vi "Insert Case Structure.vi"(0 "Custom Type Test Executive in":refnum<class "Custom Type Test Executive.lvclass">, 1 "Name":string, 2 "Unique ID":string, 3 "Insertion Index":i32=-1, 4 "Assertions":refnum<class "Assert.lvclass">[](array[class]), 5 "error in (no error)":errorcluster, 6 "Parent ID":string, 7 "X Variables":string[](array[string]), 9 "Y Variables":string[](array[string]), 11 "Conditional Branches":string[](array[string]), 13 "\"Else\" Conditional Branch":string) -> (12 "Unique ID out":string, 14 "Custom Type Test Executive out":refnum<class "Custom Type Test Executive.lvclass">, 17 "Replaced?":bool, 19 "error out":errorcluster)   [LabVIEW 2017, in "Custom Type Test Executive.lvlib" / "Custom Type Test Executive.lvclass"]
uses:
  <vilib>/gpm_packages/@cs/test-executive/Source/Custom Type Test Executive/Custom Type Test Executive/Custom Type Test Executive.lvclass
  C:/Program Files/National Instruments/LabVIEW 2017/vi.lib/gpm_packages/@cs/test-executive/Source/Test Executive/TestExecutive/Test Executive.lvclass
  <vilib>/gpm_packages/@cs/run-time-assertions/Source/Assert/Assert.lvclass
  <vilib>/gpm_packages/@cs/test-executive/Source/Custom Type Test Executive/Case Structure/Case Structure.lvclass
  <vilib>/gpm_packages/@cs/data-type-serializer/source/I32/I32.lvclass/I32.ctl
  <vilib>/gpm_packages/@cs/data-type-serializer/source/Boolean/Boolean.lvclass/Boolean.ctl
  <vilib>/gpm_packages/@cs/test-executive/Source/Test Executive/TestExecutive/Test Executive.lvclass/Test Executive.ctl
  <vilib>/gpm_packages/@cs/data-type-serializer/source/String 1D/String 1D.lvclass/String 1D.ctl
  <vilib>/gpm_packages/@cs/data-type-serializer/source/Assertion 1D/Assertion 1D.lvclass/Assertion 1D.ctl
  <vilib>/gpm_packages/@cs/data-type-serializer/source/String/String.lvclass/String.ctl
  a9862942-6bcc-4297-8062-ded843aa0e3e.vi
  f111b730-334b-4c51-af02-4347af488b46.vi
  cb5dc6a4-4407-49fc-b22c-1a23020fa038.vi
  5ed2cf76-4d61-4079-ad61-c8732e7cce71.vi
  5ea85d52-ce01-4b8a-819c-f0f3d244220a.vi
  3dbbcc80-fe4b-4aaf-9db7-d8ec31dae2ca.vi
  8353aa7f-a856-40a3-8e40-fb73858b1775.vi
  <vilib>/gpm_packages/@cs/data-type-serializer/source/String 1D/String 1D.lvclass
  <vilib>/gpm_packages/@cs/data-type-serializer/source/Assertion 1D/Assertion 1D.lvclass
  <vilib>/gpm_packages/@cs/data-type-serializer/source/String/String.lvclass
  <vilib>/gpm_packages/@cs/data-type-serializer/source/Boolean/Boolean.lvclass
  <vilib>/gpm_packages/@cs/data-type-serializer/source/I32/I32.lvclass
  <vilib>/gpm_packages/@cs/linked-list/Source/Linked List/ILinkedList/ILinked List.lvclass
  <vilib>/gpm_packages/@cs/linked-list/Source/Linked List/Linked List Ref/Linked List Ref.lvclass
  <vilib>/gpm_packages/@cs/test-executive/Source/Test Executive/TestExecutive/Test Executive.lvclass
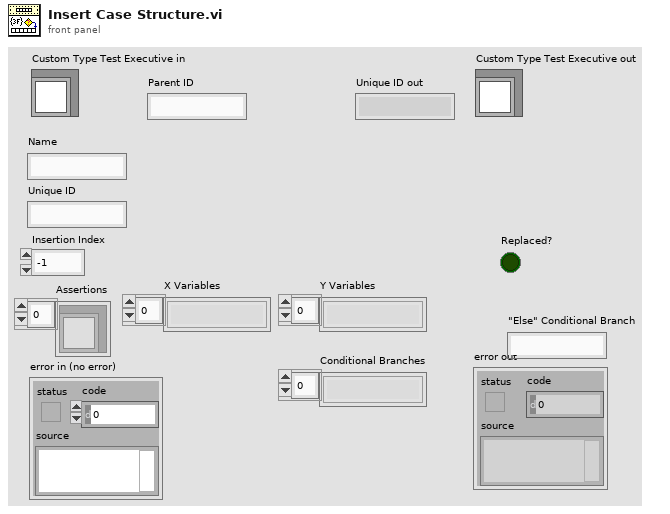
[diagram p1: front panel]
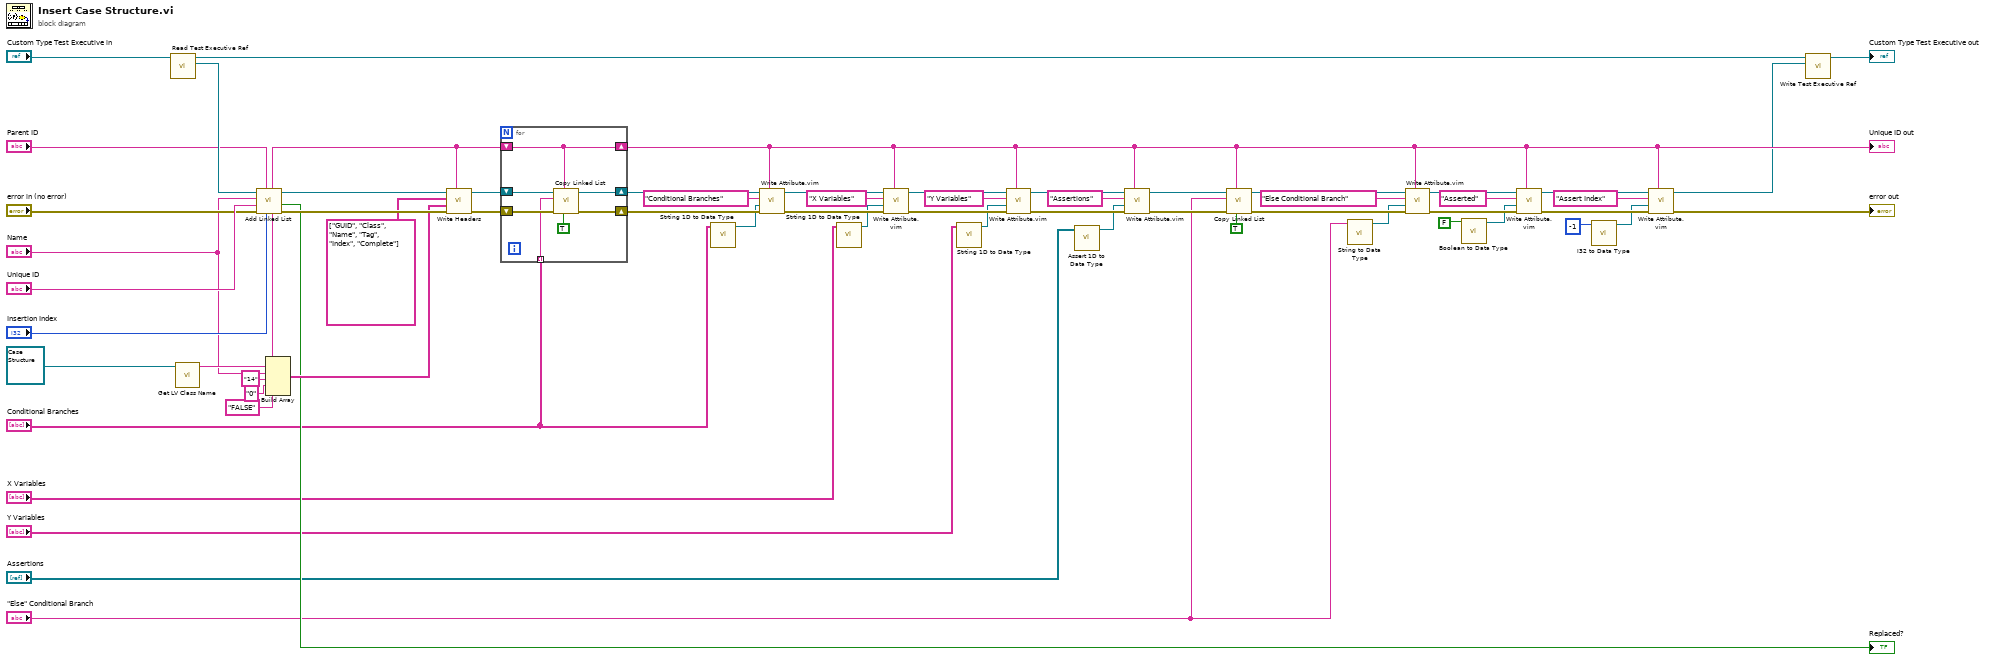
[diagram p0: block diagram]
diagram:
  n1 = call <vilib>:"Read Test Executive Ref.vi"("Test Executive in"="Custom Type Test Executive in") -> ("Test Executive Ref"=w24:refnum<data-value>, "Test Executive out"=w23:refnum<class "Custom Type Test Executive.lvclass">)  [unwired: 9 in]
  n2 = call <vilib>:"Get LV Class Name.vi"("object"=refnum<class "Case Structure.lvclass"> refnum ("Custom Type Test Executive.lvlib:Case Structure.lvclass")) -> ("class name"=w60:string)  [unwired: 9 in, 1 out]
  n3 = call <vilib>:"Add Linked List.vi"("Insertion Index"="Insertion Index", "Parent ID"="Parent ID", "error in (no error)"="error in (no error)", "Linked List ID"="Unique ID", "Name"="Name", "Linked List Ref"=w24) -> ("error out"=w62:errorcluster, "Replaced?"=→"Replaced?":bool, "Linked List Ref out"=w63:refnum<data-value>, "Linked List ID out"=w41:string)  [unwired: 2 in]
  n4 = Build Array(w41, w60, "Name", "14" ("element"), "0" ("element"), "FALSE" ("element")) -> (w58:string[])
  n5 = call <vilib>:"Write Headers.vi"("Linked List ID"=w41, "error in (no error)"=w62, "Header Values"=w58, "Header Names"=string[] ["GUID", "Class", "Name", "Tag", "Index", "Complete"], "Linked List Ref"=w63) -> ("error out"=w56:errorcluster, "Linked List Ref out"=w57:refnum<data-value>)  [unwired: 5 in]
  n6 = for {
    tunnel: "Conditional Branches" -> [w65] mode=indexing
    shift-right: [w67] -> w40
    shift-left: w57 -> [w70]
    shift-right: [w66] -> w39
    shift-left: w56 -> [w69]
    shift-right: [w64] -> w27
    shift-left: w41 -> [w64]
    n7 = call <vilib>:"Copy Linked List.vi"("Move?"=TRUE, "New Parent Linked List ID"=w64, "error in (no error)"=w69, "Linked List ID"=w65, "Linked List Ref"=w70) -> ("error out"=w66:errorcluster, "Linked List Ref out"=w67:refnum<data-value>)  [unwired: 3 in, 2 out]
  }
  "Unique ID out" <- w27
  n8 = call <vilib>:"Strting 1D to Data Type.vi"("String 1D"="Conditional Branches") -> ("Boolean out"=w13:refnum<class "String 1D.lvclass">)  [unwired: 9 in, 1 out]
  n9 = call "Write Attribute.vim"("Linked List ID"=w27, "error in (no error)"=w39, "Attribute"=w13, "Attribute Name"="Conditional Branches", "Linked List Ref"=w40) -> ("error out"=w37:errorcluster, "Linked List Ref out"=w38:refnum<data-value>)  [unwired: 3 in, 2 out]
  n10 = call <vilib>:"Strting 1D to Data Type.vi"("String 1D"="X Variables") -> ("Boolean out"=w11:refnum<class "String 1D.lvclass">)  [unwired: 9 in, 1 out]
  n11 = call "Write Attribute.vim"("Linked List ID"=w27, "error in (no error)"=w37, "Attribute"=w11, "Attribute Name"="X Variables", "Linked List Ref"=w38) -> ("error out"=w52:errorcluster, "Linked List Ref out"=w53:refnum<data-value>)  [unwired: 3 in, 2 out]
  n12 = call <vilib>:"Strting 1D to Data Type.vi"("String 1D"="Y Variables") -> ("Boolean out"=w9:refnum<class "String 1D.lvclass">)  [unwired: 9 in, 1 out]
  n13 = call "Write Attribute.vim"("Linked List ID"=w27, "error in (no error)"=w52, "Attribute"=w9, "Attribute Name"="Y Variables", "Linked List Ref"=w53) -> ("error out"=w49:errorcluster, "Linked List Ref out"=w50:refnum<data-value>)  [unwired: 3 in, 2 out]
  n14 = call <vilib>:"Assert 1D to Data Type.vi"("Assert 1D"="Assertions") -> ("Boolean out"=w7:refnum<class "Assertion 1D.lvclass">)  [unwired: 9 in, 1 out]
  n15 = call "Write Attribute.vim"("Linked List ID"=w27, "error in (no error)"=w49, "Attribute"=w7, "Attribute Name"="Assertions", "Linked List Ref"=w50) -> ("error out"=w30:errorcluster, "Linked List Ref out"=w32:refnum<data-value>)  [unwired: 3 in, 2 out]
  n16 = call <vilib>:"Copy Linked List.vi"("Move?"=TRUE, "New Parent Linked List ID"=w27, "error in (no error)"=w30, "Linked List ID"="\"Else\" Conditional Branch", "Linked List Ref"=w32) -> ("error out"=w29:errorcluster, "Linked List Ref out"=w31:refnum<data-value>)  [unwired: 3 in, 2 out]
  n17 = call <vilib>:"String to Data Type.vi"("String"="\"Else\" Conditional Branch") -> ("Boolean out"=w5:refnum<class "String.lvclass">)  [unwired: 9 in, 1 out]
  n18 = call "Write Attribute.vim"("Linked List ID"=w27, "error in (no error)"=w29, "Attribute"=w5, "Attribute Name"="Else Conditional Branch", "Linked List Ref"=w31) -> ("error out"=w35:errorcluster, "Linked List Ref out"=w36:refnum<data-value>)  [unwired: 3 in, 2 out]
  n19 = call <vilib>:"Boolean to Data Type.vi"("Boolean"=FALSE) -> ("Boolean out"=w3:refnum<class "Boolean.lvclass">)  [unwired: 9 in, 1 out]
  n20 = call "Write Attribute.vim"("Linked List ID"=w27, "error in (no error)"=w35, "Attribute"=w3, "Attribute Name"="Asserted", "Linked List Ref"=w36) -> ("error out"=w45:errorcluster, "Linked List Ref out"=w46:refnum<data-value>)  [unwired: 3 in, 2 out]
  n21 = call <vilib>:"I32 to Data Type.vi"("I32"=-1) -> ("Boolean out"=w1:refnum<class "I32.lvclass">)  [unwired: 9 in, 1 out]
  n22 = call "Write Attribute.vim"("Linked List ID"=w27, "error in (no error)"=w45, "Attribute"=w1, "Attribute Name"="Assert Index", "Linked List Ref"=w46) -> ("error out"=→"error out":errorcluster, "Linked List Ref out"=w22:refnum<data-value>)  [unwired: 3 in, 2 out]
  n23 = call <vilib>:"Write Test Executive Ref.vi"("Test Executive Ref"=w22, "Test Executive in"=w23) -> ("Test Executive out"=→"Custom Type Test Executive out":refnum<class "Custom Type Test Executive.lvclass">)  [unwired: 9 in]
